vi "Work Position.vi"(8 "Working Position":T1, 9 "Noise":dbl[](array[numeric]), 10 "A\\B":dbl[](array[numeric]), 11 "S":dbl[](array[numeric])) -> (0 "A\\B_2nd_part":dbl[](array[numeric]), 1 "S_2nd_part":dbl[](array[numeric]), 2 "A\\B_1st_part":dbl[](array[numeric]), 3 "S_1st_part":dbl[](array[numeric]), 4 "Noise_2nd_part":dbl[](array[numeric]), 5 "Noise_1st_part":dbl[](array[numeric]))   [LabVIEW 2015, in "Boimetry Processing.lvlib"]
doc: "轴向扫描信号分离。"
uses:
  Boimetry Processing.lvlib
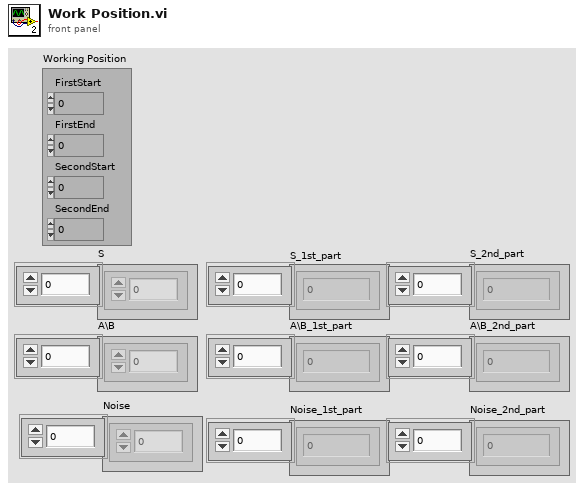
[diagram p1: front panel]
types:
  T1 = cluster{"FirstStart":i32, "FirstEnd":i32, "SecondStart":i32, "SecondEnd":i32}
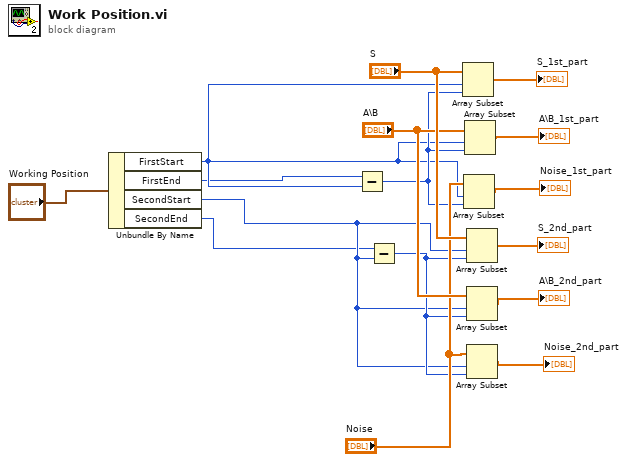
[diagram p0: block diagram]
diagram:
  n1 = Unbundle By Name("Working Position") -> ("FirstStart"=w4:i32, "FirstEnd"=w3:i32, "SecondStart"=w2:i32, "SecondEnd"=w1:i32)
  n2 = Subtract(x=w3, y=w4) -> (x-y=w9:i32)
  n3 = Subtract(x=w1, y=w2) -> (x-y=w8:i32)
  n4 = Array Subset(array="S", index=w4, length=w9) -> (→"S_1st_part":dbl[])
  n5 = Array Subset(array="Noise", index=w4, length=w9) -> (→"Noise_1st_part":dbl[])
  n6 = Array Subset(array="A\\B", index=w4, length=w9) -> (→"A\\B_1st_part":dbl[])
  n7 = Array Subset(array="S", index=w2, length=w8) -> (→"S_2nd_part":dbl[])
  n8 = Array Subset(array="A\\B", index=w2, length=w8) -> (→"A\\B_2nd_part":dbl[])
  n9 = Array Subset(array="Noise", index=w2, length=w8) -> (→"Noise_2nd_part":dbl[])
